vi "Software Initialization.vi"(8 "error in":errorcluster) -> (0 "error out":errorcluster, 2 "Events":T1)   [LabVIEW 2020]
doc: "Initialize all the software mission critical modules.\n\n-----\nJuan Navarro\nLab it Studio"
uses:
  Type Definitions/Events.ctl
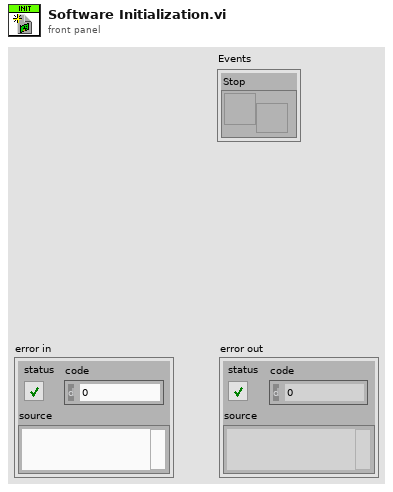
[diagram p1: front panel]
types:
  T1 = typedef "Events.ctl" = cluster{"Stop":refnum<user-event>}
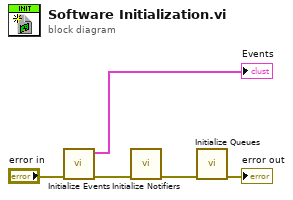
[diagram p0: block diagram]
diagram:
  n1 = call "Initialize Events.vi"("error in"="error in") -> ("error out"=w1:errorcluster, "Events"=→"Events":T1)  [unwired: 9 in]
  n2 = call "Initialize Notifiers.vi"("error in"=w1) -> ("error out"=w2:errorcluster)  [unwired: 10 in]
  n3 = call "Initialize Queues.vi"("error in"=w2) -> ("error out"=→"error out":errorcluster)  [unwired: 10 in]
